vi "FullAdder.vi"(9 "c":bool, 10 "b":bool, 11 "a":bool) -> (2 "carry":bool, 3 "sum":bool)   [LabVIEW 2014]
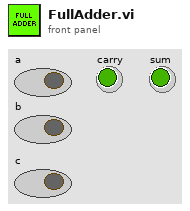
[diagram p1: front panel]
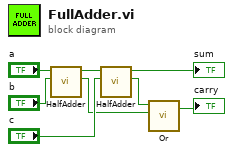
[diagram p0: block diagram]
diagram:
  n1 = call "HalfAdder.vi"("b"="b", "a"="a") -> ("carry"=w2:bool, "sum"=w6:bool)  [unwired: 8 in]
  n2 = call "HalfAdder.vi"("b"="c", "a"=w6) -> ("carry"=w3:bool, "sum"=→"sum":bool)  [unwired: 8 in]
  n3 = call "Or.vi"("b"=w2, "a"=w3) -> ("out"=→"carry":bool)  [unwired: 3 in]
